vi "Auto Intake.vi"(9 "openGear":dbl, 10 "Fill Hopper?":dbl, 11 "Roller Power":dbl) -> ()   [LabVIEW 2016]
uses:
  Common Code/Intake Modes.ctl
  Robot Global Data.vi
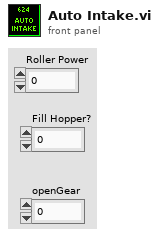
[diagram p1: front panel]
types:
  T1 = typedef "Intake Modes.ctl" = enum16{"Manual", "Auto"}
  T2 = typedef "Intake Control Cluster.ctl" = cluster{"Intake Mode":T1, "Intake Auto Command":T3, "Intake Current Trip State":T4, "Gear slot open?":bool, "Engage traction for gear load?":bool, "Wings open?":bool}
  T3 = typedef "Intake Auto States.ctl" = enum16{"Outake Ball", "Idle", "Load Ball"}
  T4 = typedef "Intake Trip States.ctl" = enum16{"Normal", "Backward Tripped", "Forward Tripped"}
  T5 = typedef "Manual Command Cluster.ctl" = cluster{"Intake Power":dbl}
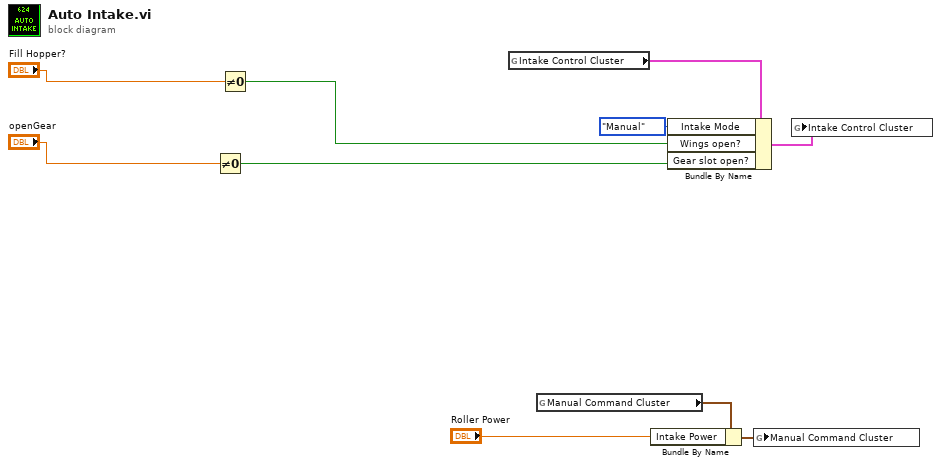
[diagram p0: block diagram]
diagram:
  n1 = Not Equal To 0?(x="openGear") -> (x != 0?=w1:bool)
  n2 = Not Equal To 0?(x="Fill Hopper?") -> (x != 0?=w3:bool)
  n3 = global read "Robot Global Data.vi" "Intake Control Cluster"() -> (w7:T2)
  n4 = global read "Robot Global Data.vi" "Manual Command Cluster"() -> (w9:T5)
  n5 = Bundle By Name(cluster=w9, "Intake Power"="Roller Power") -> (w10:T5)
  n6 = Bundle By Name(cluster=w7, "Intake Mode"=Intake_Modes."Manual", "Wings open?"=w3, "Gear slot open?"=w1) -> (w6:T2)
  n7 = global write "Robot Global Data.vi" "Manual Command Cluster"(w10) -> ()
  n8 = global write "Robot Global Data.vi" "Intake Control Cluster"(w6) -> ()
